vi "Support_SetError.vi"(1 "status":bool, 2 "code (5000)":i32=5000, 3 "source":string, 5 "error in (no error)":errorcluster) -> (19 "error out":errorcluster)   [LabVIEW 2017]
doc: "You can use this VI to generate errors."
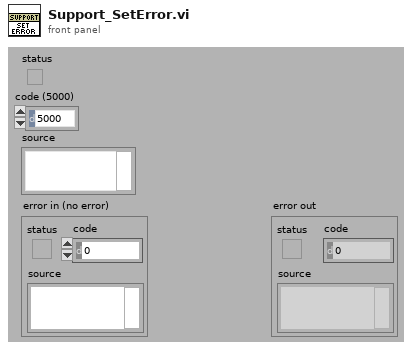
[diagram p1: front panel]
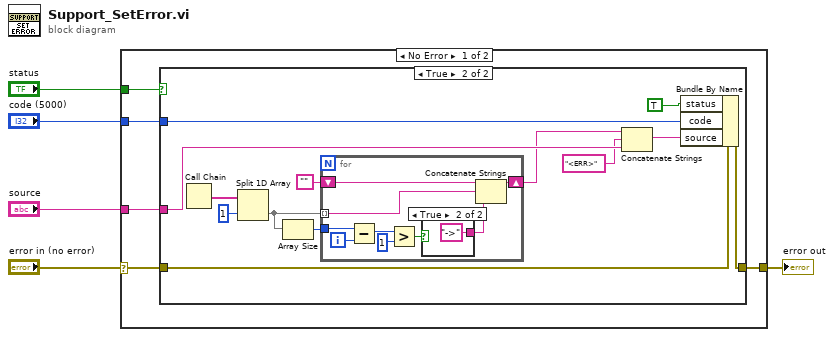
[diagram p0: block diagram]
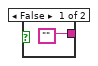
[diagram p3: hidden frame]
diagram:
  n1 = case shown="No Error" "error in (no error)" {
    selector: "error in (no error)" -> [w6 w36]
    tunnel: [w10 w36] -> w5
    tunnel: "status" -> [w9 _]
    tunnel: "code (5000)" -> [w8 _]
    tunnel: "source" -> [w7 _]
    frame No Error {
      n2 = case shown="True" w9 {
        tunnel: w6 -> [w11 w24]
        tunnel: [w11 w23] -> w10
        tunnel: w8 -> [_ w17]
        tunnel: w7 -> [_ w16]
        frame False {
        }
        frame True {
          n3 = Call Chain() -> (call chain=w21:string[])
          n4 = Split 1D Array(array=w21, index=1) -> (second subarray=w19:string[])  [unwired: 1 out]
          n5 = Array Size(array=w19) -> (size(s)=w18:i32)
          n6 = for {
            shift-right: [w25] -> w13
            shift-left: "" -> [w28]
            tunnel: w19 -> [w26] mode=indexing
            tunnel: w18 -> [w33]
            i -> [w32]
            n7 = Subtract(x=w33, y=w32) -> (x-y=w31:i32)
            n8 = Greater?(x=w31, y=1) -> (0:w29:bool)
            n9 = case shown="True" w29 {
              tunnel: ["" "->"] -> w27
              frame False {
              }
              frame True {
              }
            }
            n10 = Concatenate Strings(w28, w26, w27) -> (w25:string)
          }
          n11 = Concatenate Strings(w13, "<ERR>" ("Substring"), w16) -> (w12:string)
          n12 = Bundle By Name(cluster=w24, "status"=TRUE ("Bundle Element"), "code"=w17, "source"=w12) -> (w23:errorcluster)
        }
      }
    }
    frame Error {
    }
  }
  "error out" <- w5
